vi "Linker.Find Tests and Suites.vi"(11 "Linker:Read Info From File":T2(array[cluster])) -> (1 "All VIs defining a Test Runner":path[](array[path]), 2 "All VIs defining a suite":path[](array[path]), 3 "All VIs defining a test (excluding those defining a suite)":path[](array[path]))   [LabVIEW 2013, in "Caraya.lvlib" / "Test Runner.lvclass"]
uses:
  Test Runner.lvclass
  <vilib>/Utility/lvfile.llb/LVFileType.ctl
  <vilib>/Utility/lvfile.llb/NI_FileType.lvlib
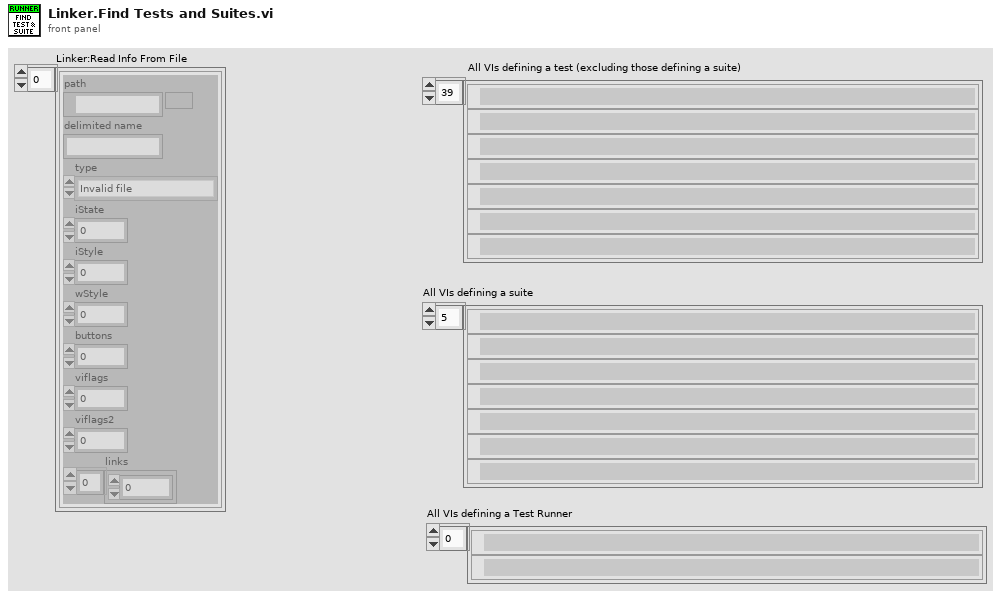
[diagram p1: front panel]
types:
  T1 = typedef "NI_FileType.lvlib/LVFileType.ctl" = enum32{"Invalid file", "Unknown type", "Instrument", "Control", "Polymorphic VI", "Project", "Library", "LVClass", "XControl", "XNode", "Shared library", ".NET assembly", "ActiveX interface", "CIN", "Run-time menu", "Palette menu", "Help file", "LLB", "XNode Edit Dependency", "Class Private Data Control", "Statechart", "MathScript .m file", "Ladder Diagram", "LVLibp", "XNode Build Dependency"}
  T2 = cluster{"path":path, "delimited name":string, "type":T1, "iState":u32, "iStyle":u16, "wStyle":u16, "buttons":u16, "viflags":u32, "viflags2":u32, "links":u32[]}[]
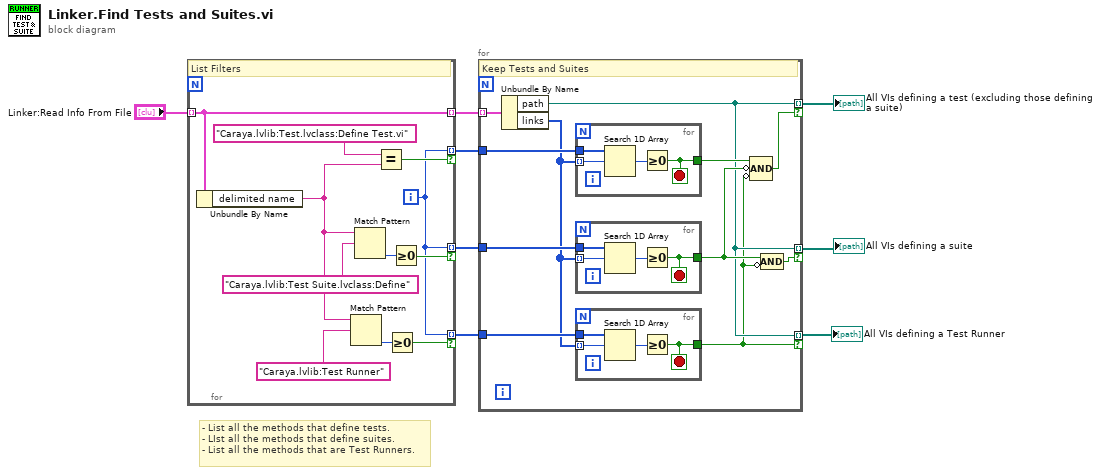
[diagram p0: block diagram]
diagram:
  # "- List all the methods that define tests.\n- LIst all the methods that define suites.\n- List all the methods that are Test Runners."
  n1 = for {
    tunnel: "Linker:Read Info From File" -> [w16] mode=indexing
    tunnel: [w10] -> w8 mode=indexing if=w18
    tunnel: [w10] -> w7 mode=indexing if=w17
    tunnel: [w16] -> w6 mode=indexing
    tunnel: [w10] -> w2 mode=indexing if=w9
    i -> [w10]
    # "List Filters"
    n2 = Unbundle By Name(w16) -> ("delimited name"=w11:string)
    n3 = Match Pattern(string=w11, regular expression="Caraya.lvlib:Test Runner" ("pattern")) -> (offset past match=w12:i32)  [unwired: 1 in, 3 out]
    n4 = Match Pattern(string=w11, regular expression="Caraya.lvlib:Test Suite.lvclass:Define" ("pattern")) -> (offset past match=w19:i32)  [unwired: 1 in, 3 out]
    n5 = Equal?(x="Caraya.lvlib:Test.lvclass:Define Test.vi" ("pattern"), y=w11) -> (x = y?=w18:bool)
    n6 = Greater Or Equal To 0?(x=w12) -> (x >= 0?=w9:bool)
    n7 = Greater Or Equal To 0?(x=w19) -> (x >= 0?=w17:bool)
  }
  n8 = for {
    tunnel: w6 -> [w26] mode=indexing
    tunnel: w8 -> [w30]
    tunnel: [w21] -> w4 mode=indexing if=w27
    tunnel: w7 -> [w29]
    tunnel: [w21] -> w3 mode=indexing if=w23
    tunnel: w2 -> [w25]
    tunnel: [w21] -> w1 mode=indexing if=w20
    # "Keep Tests and Suites"
    n9 = Unbundle By Name(w26) -> ("path"=w21:path, "links"=w24:u32[])
    n10 = for {
      tunnel: w30 -> [w42]
      tunnel: w24 -> [w41] mode=indexing
      tunnel: [w39] -> w28
      stop <- w39 stop-if-true
      n11 = Search 1D Array(1D array=w42, element=w41) -> (index of element=w40:i32)  [unwired: 1 in]
      n12 = Greater Or Equal To 0?(x=w40) -> (x >= 0?=w39:bool)
    }
    n13 = for {
      tunnel: w29 -> [w38]
      tunnel: w24 -> [w37] mode=indexing
      tunnel: [w35] -> w22
      stop <- w35 stop-if-true
      n14 = Search 1D Array(1D array=w38, element=w37) -> (index of element=w36:i32)  [unwired: 1 in]
      n15 = Greater Or Equal To 0?(x=w36) -> (x >= 0?=w35:bool)
    }
    n16 = for {
      tunnel: w25 -> [w34]
      tunnel: w24 -> [w33] mode=indexing
      tunnel: [w31] -> w20
      stop <- w31 stop-if-true
      n17 = Search 1D Array(1D array=w34, element=w33) -> (index of element=w32:i32)  [unwired: 1 in]
      n18 = Greater Or Equal To 0?(x=w32) -> (x >= 0?=w31:bool)
    }
    n19 = Compound Arithmetic op=AND(w28, invert w22, invert w20) -> (w27:bool)
    n20 = Compound Arithmetic op=AND(w22, invert w20) -> (w23:bool)
  }
  "All VIs defining a test (excluding those defining a suite)" <- w4
  "All VIs defining a suite" <- w3
  "All VIs defining a Test Runner" <- w1
